vi "Create Class.vi"(8 "error in (no error)":errorcluster, 11 "Coupled Message Rescripter in":refnum<class "Coupled Message Rescripter.lvclass">) -> (0 "error out":errorcluster, 3 "Coupled Message Rescripter out":refnum<class "Coupled Message Rescripter.lvclass">)   [LabVIEW 2020, in "Message Rescripter.lvlib" / "Coupled Message Rescripter.lvclass"]
uses:
  Coupled Message Rescripter.lvclass
  <vilib>/Utility/EditLVLibs/Edit LVLibs.lvlib
  Message Rescripter.lvlib
  MessageMakerProvider/_Message Maker/Message Maker.lvlib
  MessageMakerProvider/_Message Maker/_Maker Classes/Message Scripter/Message Scripter.lvclass
  <vilib>/Utility/traverseref.llb/TRef TravTarget.ctl
  MessageMakerProvider/_Message Maker/_Maker Classes/Concrete Send Builder/Concrete Send Builder.lvclass
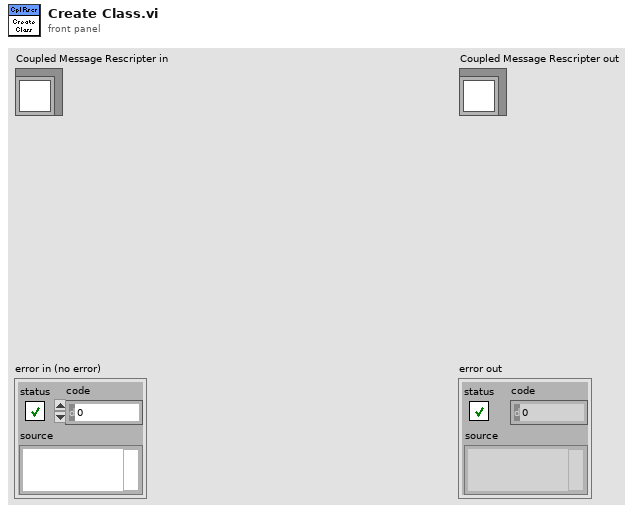
[diagram p1: front panel]
types:
  T1 = typedef "TRef TravTarget.ctl" = enum16{"FP", "BD", "Other"}
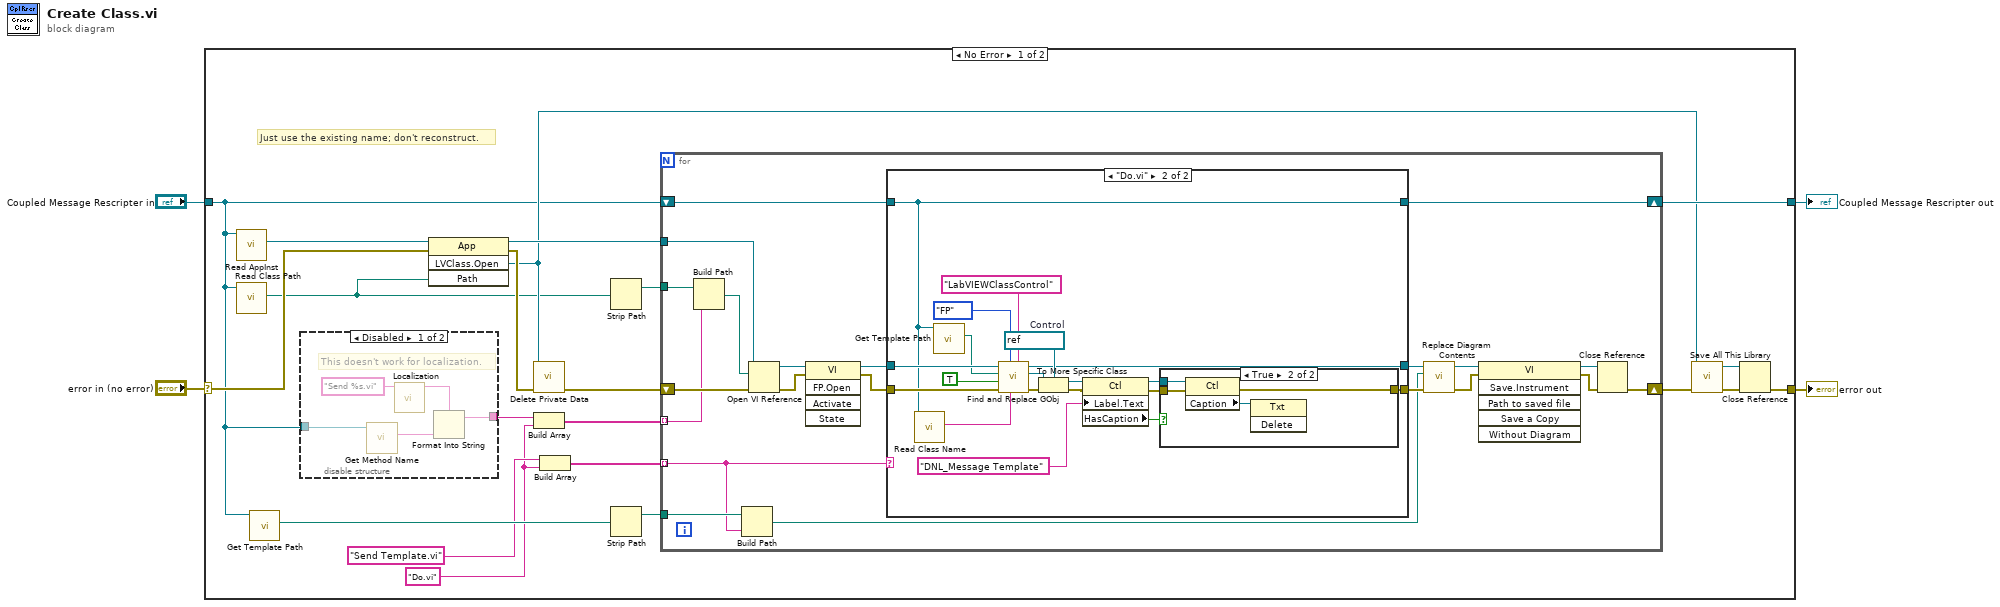
[diagram p0: block diagram]
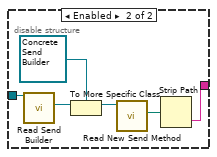
[diagram p2: hidden frame]
diagram:
  n1 = case shown="No Error" "error in (no error)" {
    selector: "error in (no error)" -> [w12 w86]
    tunnel: [w15 w86] -> w4
    tunnel: [w14 w85] -> w3
    tunnel: "Coupled Message Rescripter in" -> [w5 w85]
    frame No Error {
      w18 = "Do.vi" ("element")
      # "Just use the existing name; don't reconstruct."
      n2 = call "Read AppInst.vi"("Message Maker in"=w5) -> ("AppInst"=w9:refnum<vi>)  [unwired: 10 in]
      n3 = call "Read Class Path.vi"("Message Scripter in"=w5) -> ("Class Path"=w8:path)  [unwired: 10 in]
      n4 = call-dynamic "Get Template Path.vi"("Coupled Message Scripter in"=w5) -> ("Template Path"=w24:path)  [unwired: 10 in]
      n5 = disable-structure shown="Disabled" {
        disable-tunnel: [w28 w32] -> w17
        disable-tunnel: w5 -> [w26 w31]
        frame Disabled {
          # "This doesn't work for localization."
          n6 = call-dynamic "Get Method Name.vi"("Message Maker in"=w26) -> ("Method Name"=w27:string)  [unwired: 10 in]
          n7 = call "Localization.vi"("Unlocalized"="Send %s.vi") -> ("Localized"=w29:string)  [unwired: 10 in]
          n8 = Format Into String(format string=w29, w27) -> (resulting string=w28:string)  [unwired: 2 in, 1 out]
        }
        frame Enabled {
          n9 = call-dynamic "Read Send Builder.vi"("Message Scripter in"=w31) -> ("Send Builder"=w33:refnum<class "Send Builder.lvclass">)  [unwired: 10 in]
          n10 = To More Specific Class(target class=refnum<class "Concrete Send Builder.lvclass"> refnum ("Concrete Send Builder in"), reference=w33) -> (specific class reference=w35:refnum<class "Concrete Send Builder.lvclass">)  [unwired: 1 in, 1 out]
          n11 = call-dynamic "Read New Send Method.vi"("Concrete Send Builder in"=w35) -> ("New Send Method"=w36:path)  [unwired: 10 in]
          n12 = Strip Path(path=w36) -> (name=w32:string)  [unwired: 1 out]
        }
      }
      n13 = invoke class="App" method="LVClass.Open"(reference=w9, error in=w12, "Path"=w8) -> (reference out=w23:refnum<vi>, error out=w13:errorcluster, "LVClass.Open"=w11:refnum<vi>)  [unwired: 1 in, 1 out]
      n14 = call "Delete Private Data.vi"("error in (no error)"=w13, "LVClassLibrary in"=w11) -> ("error out"=w25:errorcluster)  [unwired: 9 in]
      n15 = Build Array(w17, w18) -> (w21:string[])
      n16 = Build Array("Send Template.vi" ("Method"), w18) -> (w19:string[])
      n17 = Strip Path(path=w8) -> (stripped path=w7:path)  [unwired: 1 out]
      n18 = Strip Path(path=w24) -> (stripped path=w6:path)  [unwired: 1 out]
      n19 = for {
        shift-right: [w52] -> w22
        shift-left: w25 -> [w55]
        tunnel: w23 -> [w57]
        tunnel: w7 -> [w51]
        tunnel: w21 -> [w54] mode=indexing
        tunnel: w6 -> [w53]
        tunnel: w19 -> [w50] mode=indexing
        shift-right: [w48] -> w14
        shift-left: w5 -> [w49]
        n20 = Build Path(base path=w51, name or relative path=w54) -> (appended path=w56:path)
        n21 = Build Path(base path=w53, name or relative path=w50) -> (appended path=w43:path)
        n22 = Open VI Reference(application reference (local)=w57, vi path=w56, error in (no error)=w55) -> (vi reference=w42:refnum<vi>, error out=w40:errorcluster)  [unwired: 3 in]
        n23 = invoke class="VI" method="FP.Open"(reference=w42, error in=w40) -> (reference out=w41:refnum<vi>, error out=w39:errorcluster)  [unwired: 3 in, 3 out]
        n24 = case shown="\"Do.vi\"" w50 {
          tunnel: w41 -> [w59 w79]
          tunnel: w39 -> [w58 w78]
          tunnel: [w60 w76] -> w48
          tunnel: w49 -> [w60 w76]
          tunnel: [w59 w63] -> w44
          tunnel: [w58 w64] -> w45
          frame "False", Default {
          }
          frame "Do.vi" {
            w71 = refnum<vi> refnum  # Control
            n25 = call "Read Class Name.vi"("Message Scripter in"=w76) -> ("Class Name"=w77:string)  [unwired: 10 in]
            n26 = call-dynamic "Get Template Path.vi"("Coupled Message Scripter in"=w76) -> ("Template Path"=w75:path)  [unwired: 10 in]
            n27 = call "Find and Replace GObj.vi"("GObj Class Name"="LabVIEWClassControl", "GObj Label"=w77, "Traverse Target"=TRef_TravTarget."FP", "error in (no error)"=w78, "Case Insensitive Match? (F)"=TRUE, "Class Path"=w75, "vi reference in"=w79) -> ("error out"=w72:errorcluster, "Replace"=w62:refnum<vi>, "vi reference out"=w63:refnum<vi>)  [unwired: 2 in]
            n28 = To More Specific Class(target class=w71, reference=w62, error in=w72) -> (specific class reference=w65:refnum<vi>, error out=w66:errorcluster)
            n29 = property class="Ctl"(reference=w65, error in=w66, "Label.Text"="DNL_Message Template") -> (reference out=w67:refnum<vi>, error out=w68:errorcluster, "HasCaption"=w69:bool)
            n30 = case shown="True" w69 {
              tunnel: w67 -> [_ w83]
              tunnel: w68 -> [w80 w82]
              tunnel: [w80 w81] -> w64
              frame False {
              }
              frame True {
                n31 = property class="Ctl"(reference=w83, error in=w82) -> (error out=w81:errorcluster, "Caption"=w84:refnum<vi>)  [unwired: 1 out]
                n32 = invoke class="Txt" method="Delete"(reference=w84) -> ()  [unwired: 2 in, 3 out]
              }
            }
          }
        }
        n33 = call "Replace Diagram Contents.vi"("error in (no error)"=w45, "Template VI"=w43, "Target VI"=w44) -> ("error out"=w46:errorcluster, "dup Target VI"=w47:refnum<vi>)  [unwired: 7 in]
        n34 = invoke class="VI" method="Save.Instrument"(reference=w47, error in=w46) -> (reference out=w38:refnum<vi>, error out=w37:errorcluster)  [unwired: 4 in, 4 out]
        n35 = Close Reference(reference=w38, error in (no error)=w37) -> (error out=w52:errorcluster)
      }
      n36 = call <vilib>:"Save All This Library.vi"("error in (no error)"=w22, "Library in"=w11) -> ("error out"=w16:errorcluster, "Library out"=w10:refnum<vi>)  [unwired: 8 in]
      n37 = Close Reference(reference=w10, error in (no error)=w16) -> (error out=w15:errorcluster)
    }
    frame Error {
    }
  }
  "error out" <- w4
  "Coupled Message Rescripter out" <- w3
